vi "停止整机测试(子VI).vi"() -> (0 "error out":T1={"status"=FALSE, "代码"=4, "source"=""} caption="错误输出" {"代码" items=["执行成功"=1, "执行失败，但不知道原因"=2, "命令请求条件错误"=3, "通讯超时"=4, "系统繁忙不能执行"=5, "系统故障"=6, "没有数据"=100]})   [LabVIEW 2016]
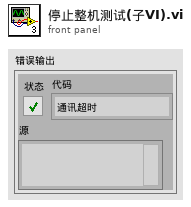
[diagram p1: front panel]
types:
  T1 = cluster{"status":bool, "代码":u16, "source":string}
  T2 = cluster{"参数启用":cluster{"氨氮":bool, "总磷":bool, "总氮":bool, "多参数":bool, "CODMn":bool, "CODcr":bool, "超标留样":bool}}
  T3 = cluster{"命令":string, cluster{"starting address":u16, "holding register value":u16}}
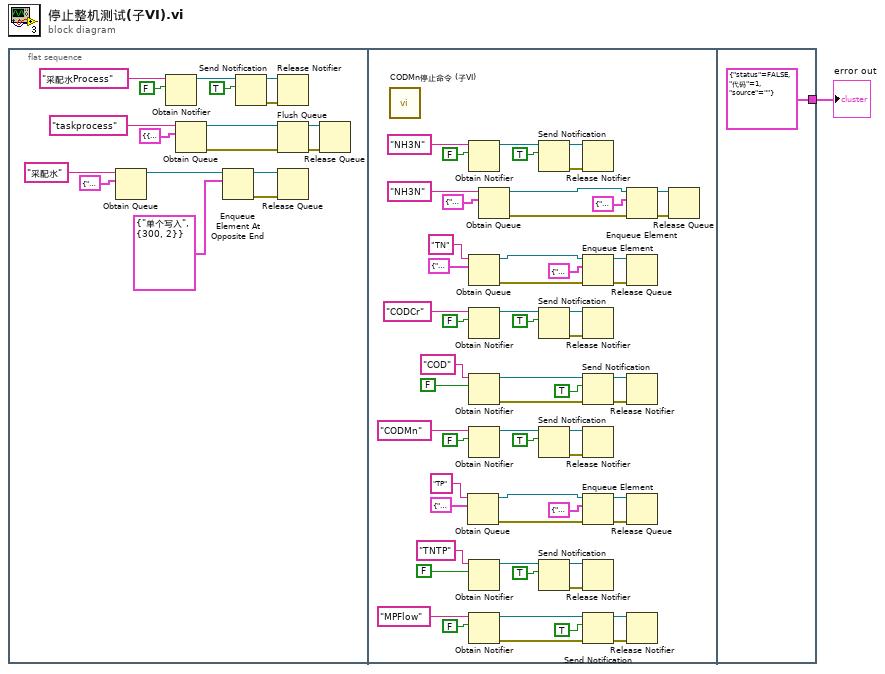
[diagram p0: block diagram]
diagram:
  n1 = flat-sequence {
    tunnel: [T1 {"status"=FALSE, "代码"=1, "source"=""} ("error out")] -> w1
    frame #0 {
      n2 = Obtain Queue(name (unnamed)="采配水" ("名称（未命名）"), element data type=cluster{"命令":string, "数据":variant} {"命令"="", "数据"=variant}) -> (queue out=w17:refnum<queue>)  [unwired: 3 in, 2 out]
      n3 = Obtain Notifier(name (unnamed)="采配水Process" ("名称（未命名）"), notification data type=FALSE) -> (notifier out=w19:refnum<notifier>)  [unwired: 2 in, 2 out]
      n4 = Obtain Queue(name (unnamed)="taskprocess" ("名称（未命名）"), element data type=T2 {"参数启用"={"氨氮"=FALSE, "总磷"=FALSE, "总氮"=FALSE, "多参数"=FALSE, "CODMn"=FALSE, "CODcr"=FALSE, "超标留样"=FALSE}} ("参数")) -> (queue out=w5:refnum<queue>, error out=w4:errorcluster)  [unwired: 3 in, 1 out]
      n5 = Enqueue Element At Opposite End(queue=w17, element=T3 {"命令"="单个写入", {"starting address"=300, "holding register value"=2}} ("元素")) -> (queue out=w11:refnum<queue>, error out=w10:errorcluster)  [unwired: 2 in, 1 out]
      n6 = Send Notification(notification=TRUE ("通知"), notifier=w19) -> (notifier out=w9:refnum<notifier>, error out=w8:errorcluster)  [unwired: 1 in]
      n7 = Release Notifier(notifier=w9, error in (no error)=w8) -> ()  [unwired: 1 in, 3 out]
      n8 = Flush Queue(queue=w5, error in (no error)=w4) -> (queue out=w2:refnum<queue>, error out=w3:errorcluster)  [unwired: 1 out]
      n9 = Release Queue(queue=w11, error in (no error)=w10) -> ()  [unwired: 1 in, 3 out]
      n10 = Release Queue(queue=w2, error in (no error)=w3) -> ()  [unwired: 1 in, 3 out]
    }
    frame #1 {
      n11 = call "CODMn停止命令 (子VI).vi"() -> ()  [unwired: 12 in]
      n12 = Obtain Queue(name (unnamed)="TP" ("名称（未命名）"), element data type=cluster{"命令":string, "data":variant} {"命令"="", "data"=variant}) -> (queue out=w71:refnum<queue>, error out=w48:errorcluster)  [unwired: 3 in, 1 out]
      n13 = Obtain Notifier(name (unnamed)="NH3N" ("名称（未命名）"), notification data type=FALSE) -> (notifier out=w75:refnum<notifier>)  [unwired: 2 in, 2 out]
      n14 = Obtain Queue(name (unnamed)="TN" ("名称（未命名）"), element data type=cluster{"命令":string, "data":variant} {"命令"="", "data"=variant}) -> (queue out=w44:refnum<queue>, error out=w43:errorcluster)  [unwired: 3 in, 1 out]
      n15 = Obtain Notifier(name (unnamed)="CODCr" ("名称（未命名）"), notification data type=FALSE) -> (notifier out=w54:refnum<notifier>)  [unwired: 2 in, 2 out]
      n16 = Obtain Notifier(name (unnamed)="COD" ("名称（未命名）"), notification data type=FALSE) -> (notifier out=w23:refnum<notifier>, error out=w24:errorcluster)  [unwired: 2 in, 1 out]
      n17 = Obtain Notifier(name (unnamed)="CODMn" ("名称（未命名）"), notification data type=FALSE) -> (notifier out=w60:refnum<notifier>)  [unwired: 2 in, 2 out]
      n18 = Obtain Notifier(name (unnamed)="TNTP" ("名称（未命名）"), notification data type=FALSE) -> (notifier out=w67:refnum<notifier>)  [unwired: 2 in, 2 out]
      n19 = Obtain Notifier(name (unnamed)="MPFlow" ("名称（未命名）"), notification data type=FALSE) -> (notifier out=w56:refnum<notifier>, error out=w55:errorcluster)  [unwired: 2 in, 1 out]
      n20 = Obtain Queue(name (unnamed)="NH3N" ("名称（未命名）"), element data type=cluster{"命令":string, "data":variant} {"命令"="", "data"=variant}) -> (queue out=w78:refnum<queue>, error out=w47:errorcluster)  [unwired: 3 in, 1 out]
      n21 = Send Notification(notification=TRUE ("通知"), notifier=w75) -> (notifier out=w36:refnum<notifier>, error out=w35:errorcluster)  [unwired: 1 in]
      n22 = Send Notification(notification=TRUE ("通知"), notifier=w54) -> (notifier out=w30:refnum<notifier>, error out=w29:errorcluster)  [unwired: 1 in]
      n23 = Send Notification(notification=TRUE ("通知"), notifier=w60) -> (notifier out=w32:refnum<notifier>, error out=w31:errorcluster)  [unwired: 1 in]
      n24 = Send Notification(notification=TRUE ("通知"), notifier=w67) -> (notifier out=w34:refnum<notifier>, error out=w33:errorcluster)  [unwired: 1 in]
      n25 = Release Notifier(notifier=w36, error in (no error)=w35) -> ()  [unwired: 1 in, 3 out]
      n26 = Enqueue Element(queue=w44, element=cluster{"命令":string, "data":variant} {"命令"="启动", "data"=variant(cluster{"站号":u16, "控制命令输出":u16[]} {"站号"=2, "控制命令输出"=[2816]})} ("元素"), error in (no error)=w43) -> (queue out=w42:refnum<queue>, error out=w41:errorcluster)  [unwired: 1 in, 1 out]
      n27 = Release Notifier(notifier=w30, error in (no error)=w29) -> ()  [unwired: 1 in, 3 out]
      n28 = Send Notification(notification=TRUE ("通知"), notifier=w23, error in (no error)=w24) -> (notifier out=w25:refnum<notifier>, error out=w26:errorcluster)
      n29 = Release Notifier(notifier=w32, error in (no error)=w31) -> ()  [unwired: 1 in, 3 out]
      n30 = Enqueue Element(queue=w71, element=cluster{"命令":string, "data":variant} {"命令"="启动", "data"=variant(cluster{"站号":u16, "控制命令输出":u16[]} {"站号"=1, "控制命令输出"=[2816]})} ("元素"), error in (no error)=w48) -> (queue out=w40:refnum<queue>, error out=w39:errorcluster)  [unwired: 1 in, 1 out]
      n31 = Release Notifier(notifier=w34, error in (no error)=w33) -> ()  [unwired: 1 in, 3 out]
      n32 = Send Notification(notification=TRUE ("通知"), notifier=w56, error in (no error)=w55) -> (notifier out=w28:refnum<notifier>, error out=w27:errorcluster)
      n33 = Enqueue Element(queue=w78, element=cluster{"命令":string, "data":variant} {"命令"="启动", "data"=variant(cluster{"站号":u16, "控制命令输出":u16[]} {"站号"=3, "控制命令输出"=[2816]})} ("启动命令"), error in (no error)=w47) -> (queue out=w38:refnum<queue>, error out=w37:errorcluster)  [unwired: 1 in, 1 out]
      n34 = Release Queue(queue=w42, error in (no error)=w41) -> ()  [unwired: 1 in, 3 out]
      n35 = Release Notifier(notifier=w25, error in (no error)=w26) -> ()  [unwired: 1 in, 3 out]
      n36 = Release Queue(queue=w40, error in (no error)=w39) -> ()  [unwired: 1 in, 3 out]
      n37 = Release Notifier(notifier=w28, error in (no error)=w27) -> ()  [unwired: 1 in, 3 out]
      n38 = Release Queue(queue=w38, error in (no error)=w37) -> ()  [unwired: 1 in, 3 out]
    }
    frame #2 {
    }
  }
  "error out" <- w1
